vi "Main.vi"(0 "Search Bar":string, 1 "Copy":bool, 2 "Expand/Collapse All":bool, 5 "Tree":string[](tree), 7 "Top Level folder path":path, 11 "Error In":errorcluster) -> (4 "Report String":string, 15 "Error Out":errorcluster)   [LabVIEW 2019]
doc: "Implements a file explorer interface to display folders and files, displaying attributes and supporting operations like selection, copying, sorting and report generation about the folders."
uses:
  Controls/Queue Operation.ctl
  Controls/Queue Element.ctl
  Controls/File explorer Data.ctl
  Controls/Item.ctl
  <vilib>/Utility/miscctls.llb/LVPoint32TypeDef.ctl
panel:
  # "Instructions:\n1. Run the VI.\n2. Specify the top-level folder path and view the folder structure along with its attributes in the tree control.\n3. Tree headers acts as sorting triggers.\n4. Click the checkbox next to folder to select or deselect it. View the generated report for the checked folders in the report string.\n5. Press the Expand/Collapse button to expand/collapse all the items in the tree.\n6. Enter the folder name in the search bar to expand all the nodes that match the searched keyword.\n7. Select the files and click on the copy to copy the files in the new folder of the desired destination.\n8. Click Panel Close to stop the VI."
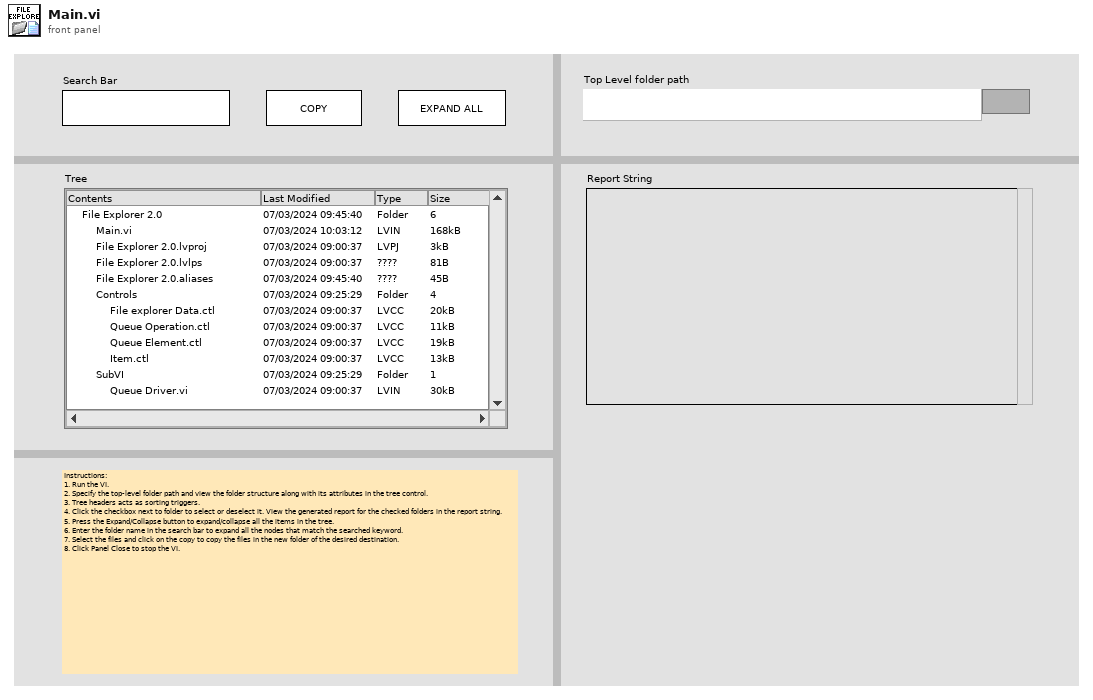
[diagram p1: front panel]
types:
  T1 = typedef "Queue Element.ctl" = cluster{"State":string, "Data":variant}
  T2 = typedef "File explorer Data.ctl" = cluster{"Path In":path, "Indent":i32, "All Folders":path[], "All Files":path[], "Folder Items":cluster{"Left Cell String":string, "Child Text":string[], "Child Tag":string, "Item Indent":i32, "Child Only?":bool, "Glyph Index":i32}[], "File Items":T3[], "Selected tags":string[], "Report String":string, "Search String":string, "Search Results":string[], "Checked Folders":string[], "Files Selected":string[], "Stop Event":refnum<user-event>, "Sort Header":i32, "Time Flag":i16, "Type Flag":i16, "Size Flag":i16, "Reverse?":bool, "New Folder Path":path, "Expand?":bool, "Open? State":bool[], "Nodes":path[]}
  T3 = typedef "Item.ctl" = cluster{"Left Cell String":string, "Child Text":string[], "Child Tag":string, "Child Only?":bool, "Parent Tag":string, "Item Indent":i32}
  T4 = typedef "Queue Operation.ctl" = enum16{"Create", "Enqueue", "Enqueue N", "Dequeue", "Enstack N", "Flush", "Release"}
  T5 = cluster{"Left Cell String":string, "Child Text":string[], "Child Tag":string, "Item Indent":i32, "Child Only?":bool, "Glyph Index":i32}
  T6 = typedef "LVPoint32TypeDef.ctl" = cluster{"Horizontal":i32, "Vertical":i32}
  T7 = cluster{"Left Cell String":string, "Child Text":string[], "Child Tag":string, "Item Indent":i32, "Child Only?":bool, "Glyph Index":i32}[]
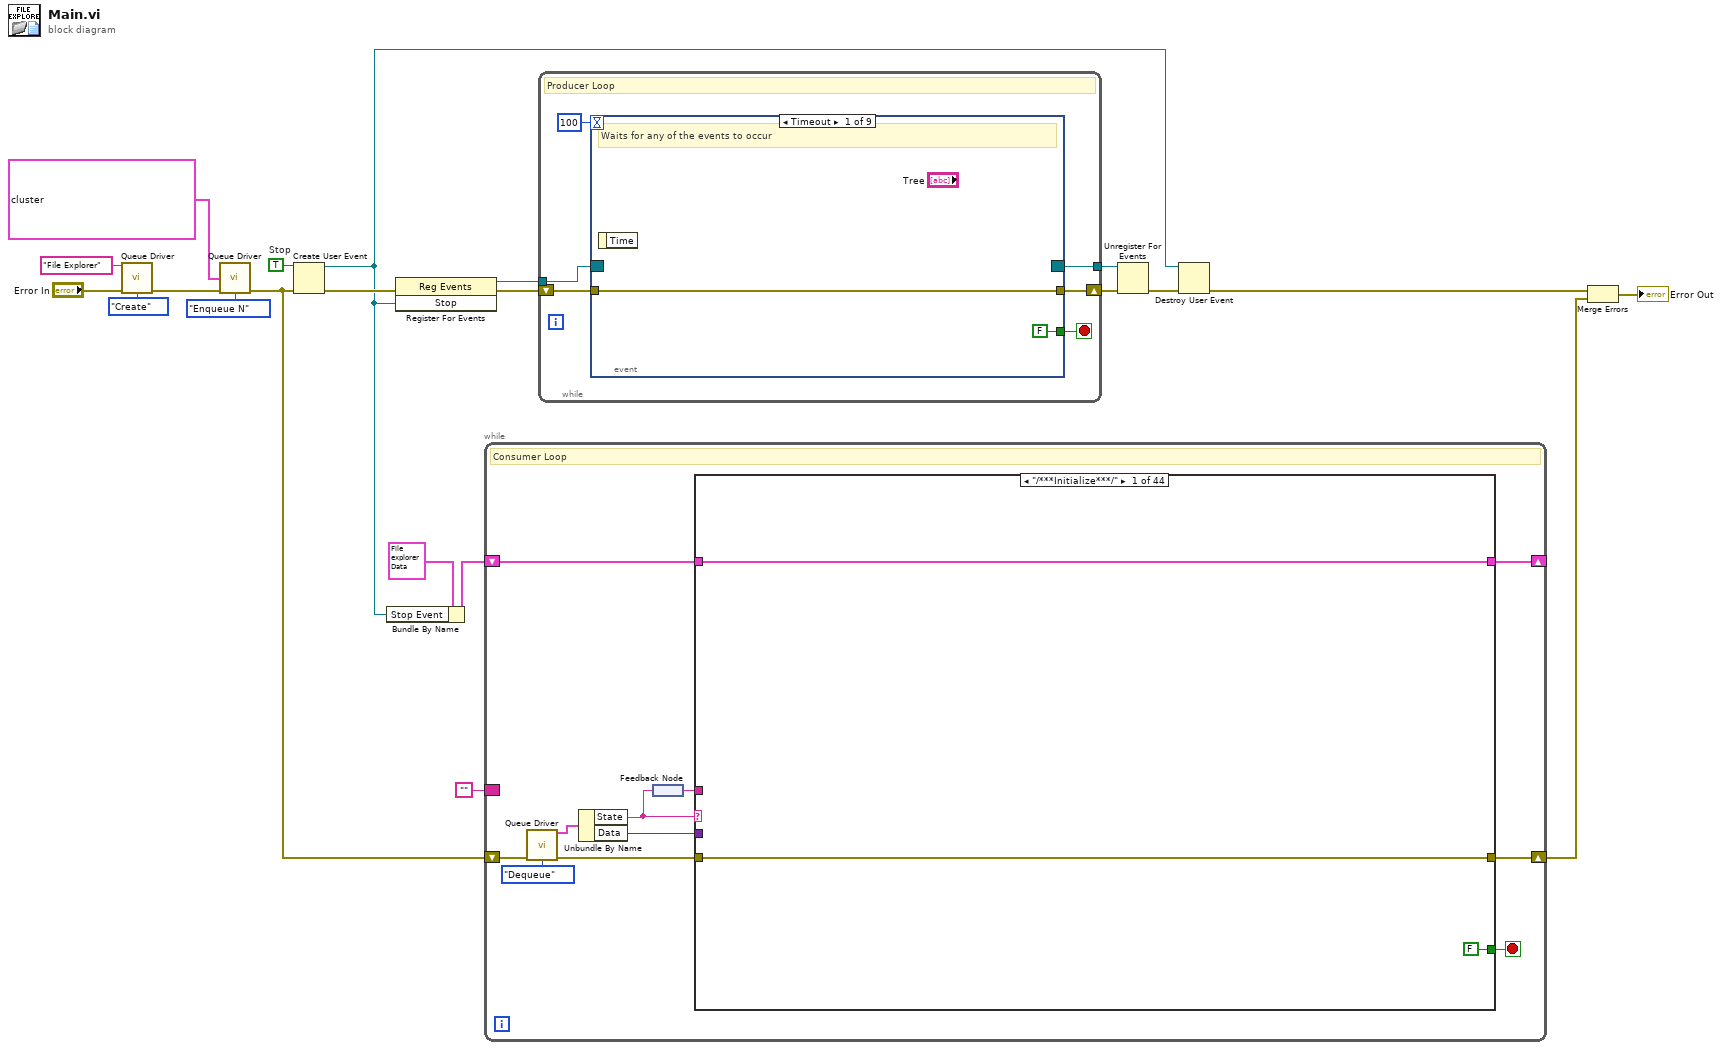
[diagram p0: block diagram]
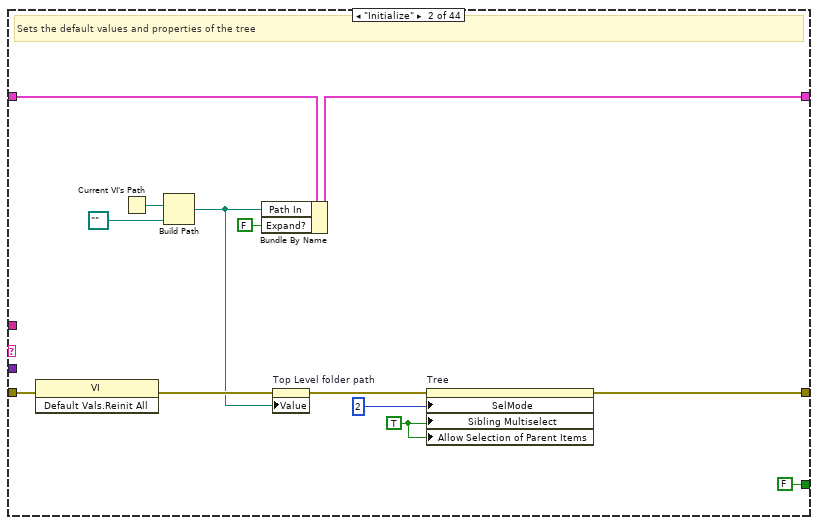
[diagram p2: hidden frame]
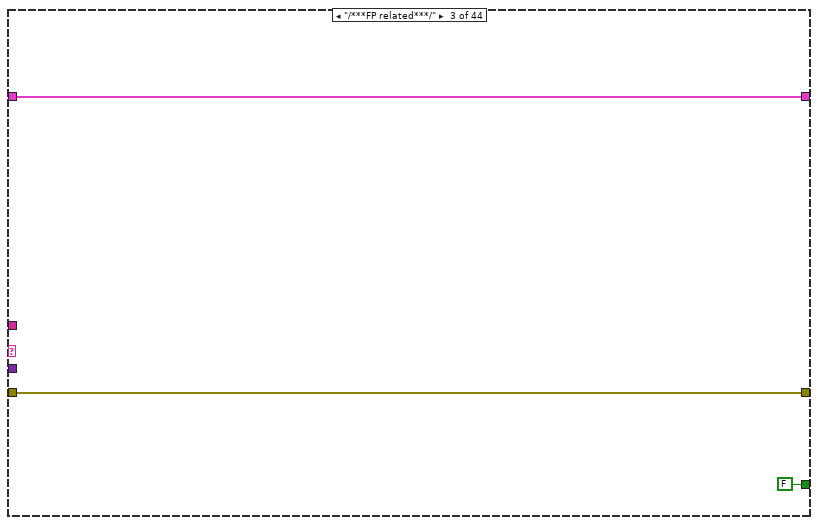
[diagram p3: hidden frame]
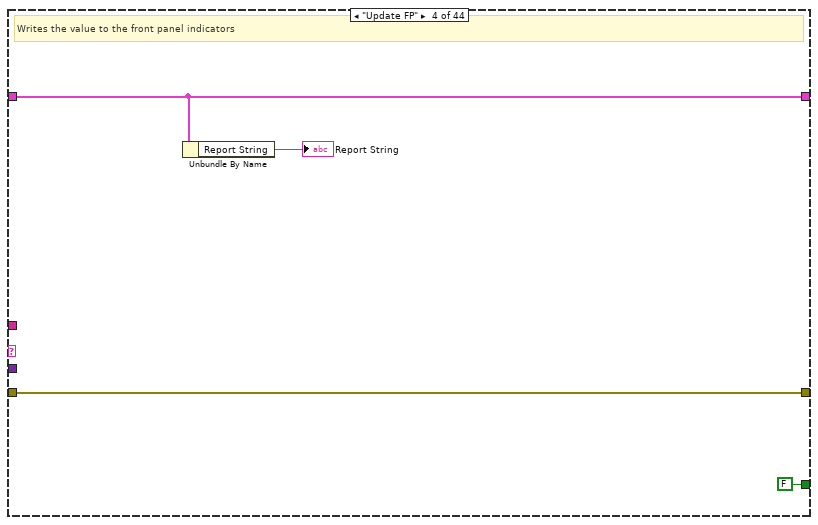
[diagram p4: hidden frame]
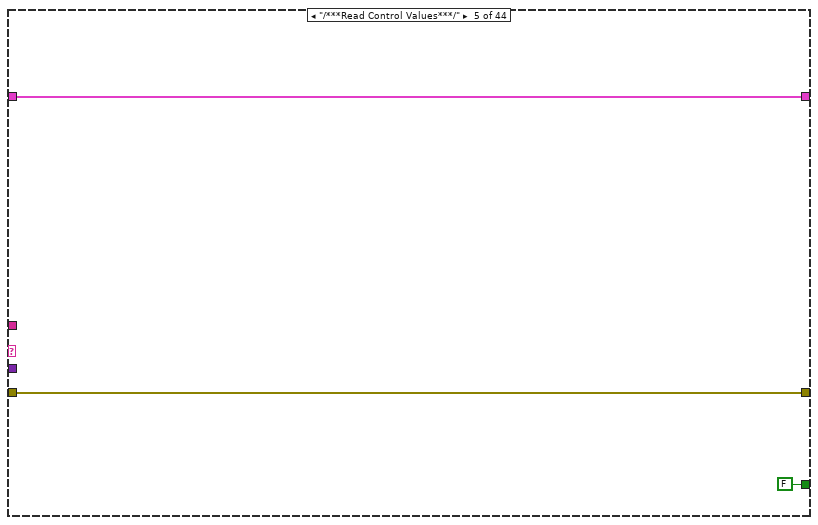
[diagram p5: hidden frame]
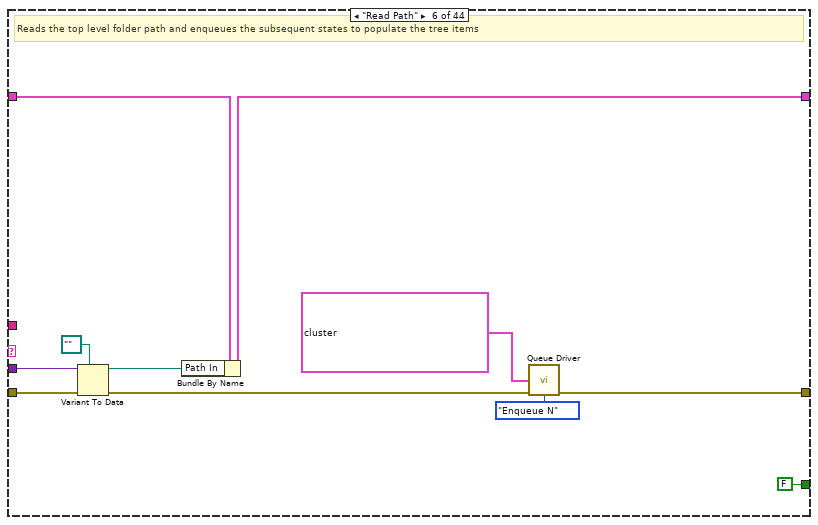
[diagram p6: hidden frame]
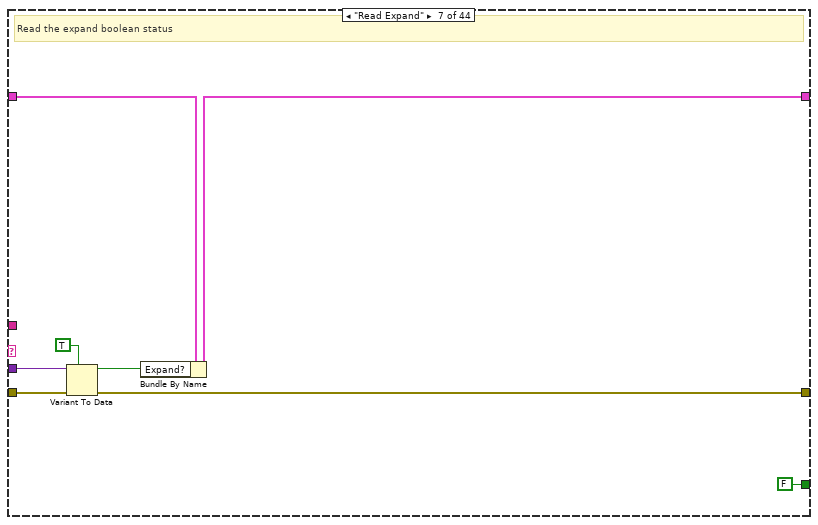
[diagram p7: hidden frame]
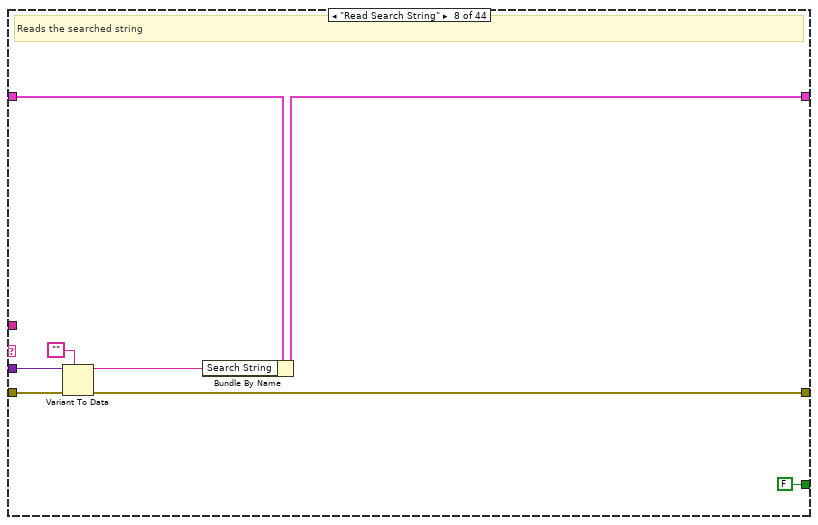
[diagram p8: hidden frame]
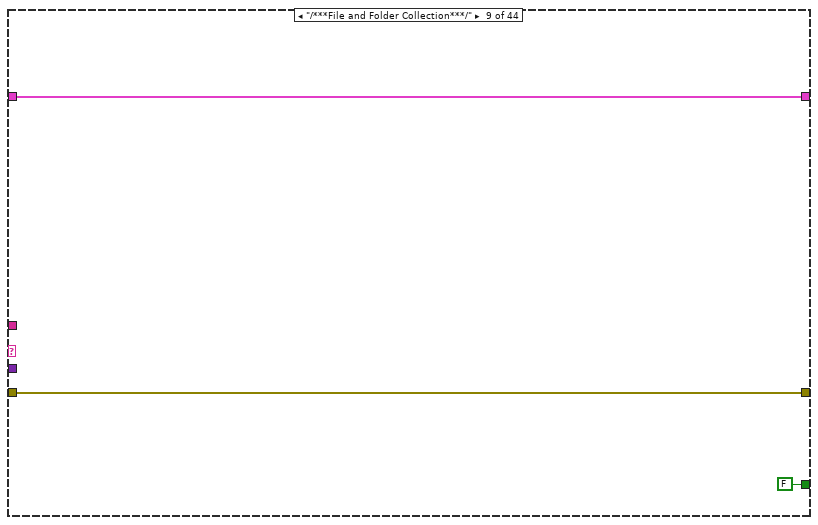
[diagram p9: hidden frame]
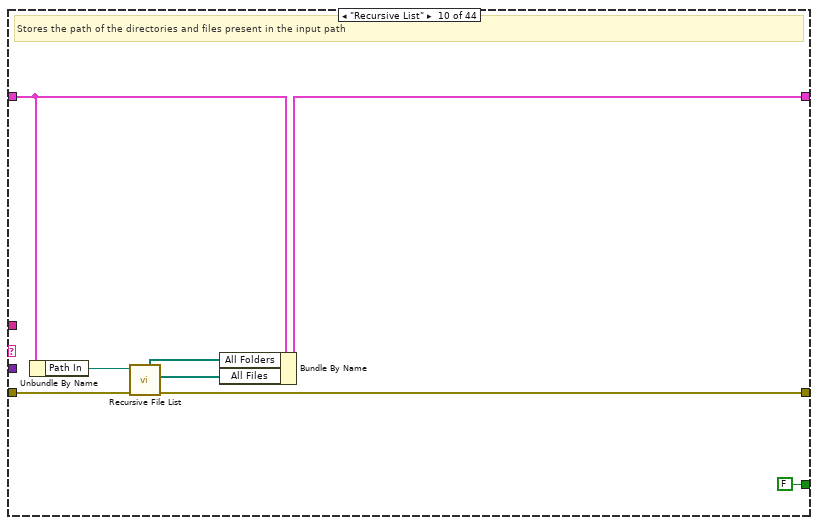
[diagram p10: hidden frame]
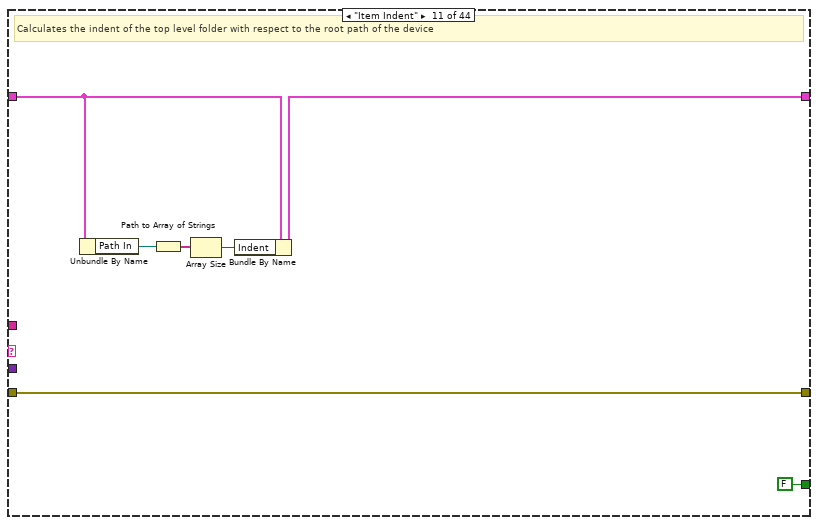
[diagram p11: hidden frame]
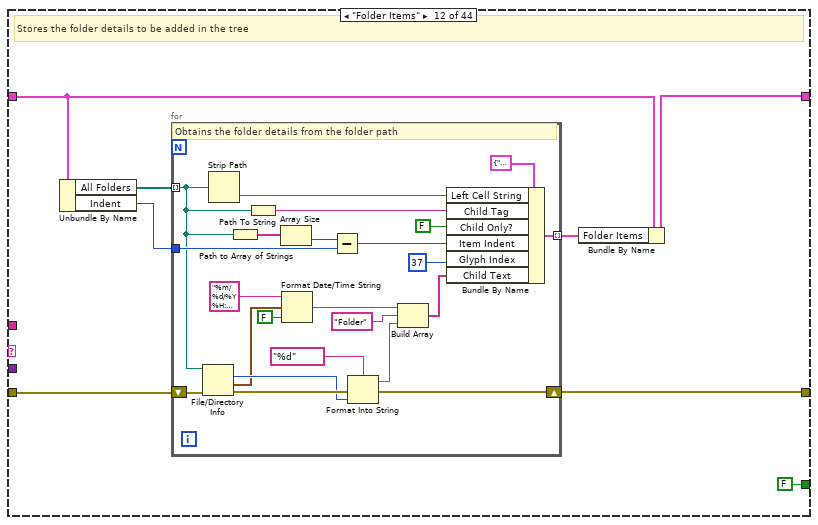
[diagram p12: hidden frame]
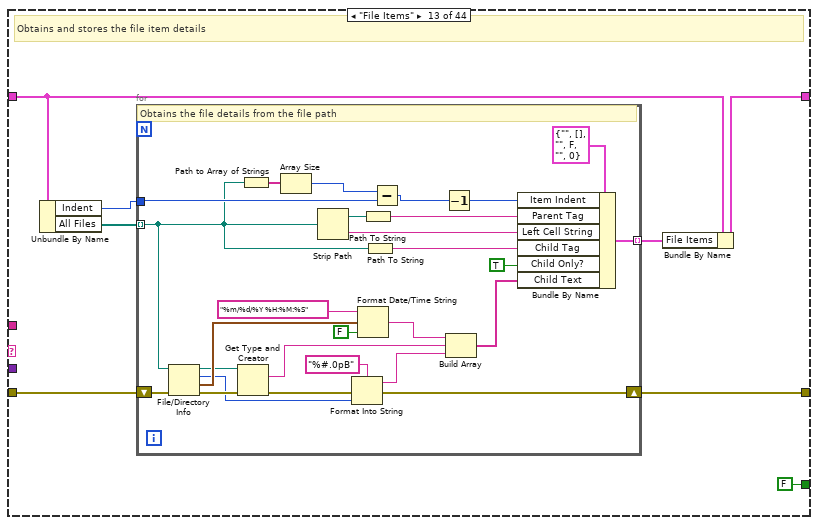
[diagram p13: hidden frame]
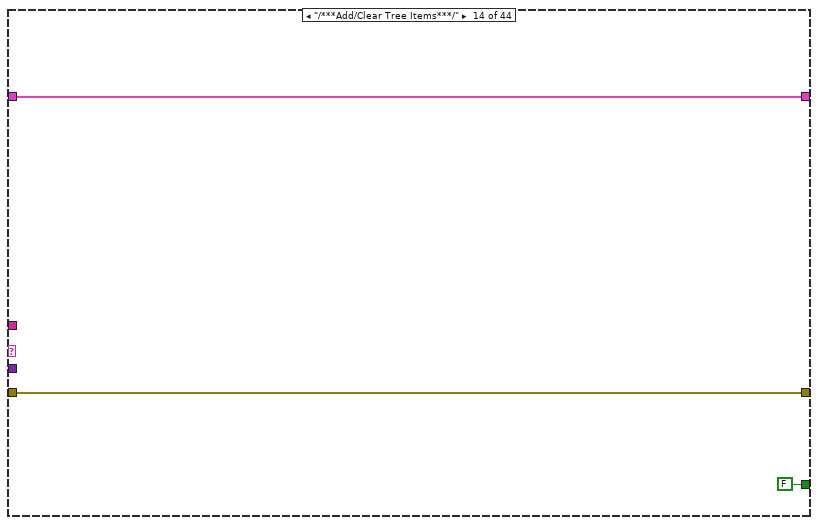
[diagram p14: hidden frame]
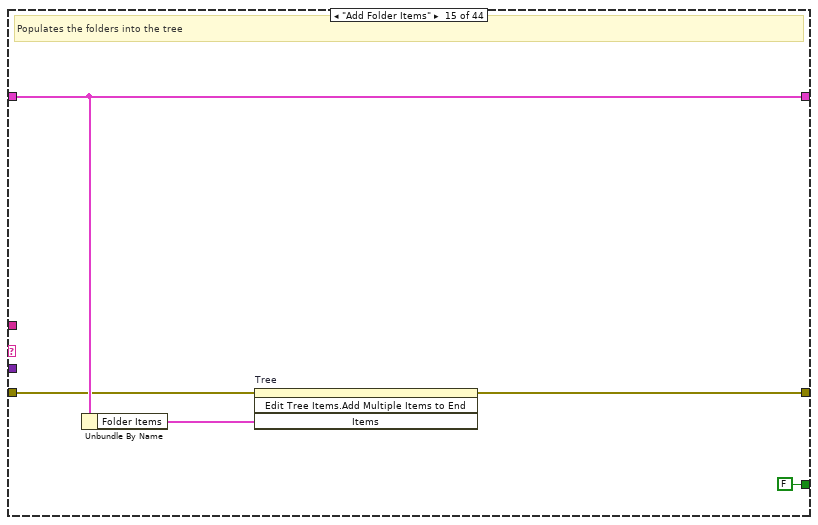
[diagram p15: hidden frame]
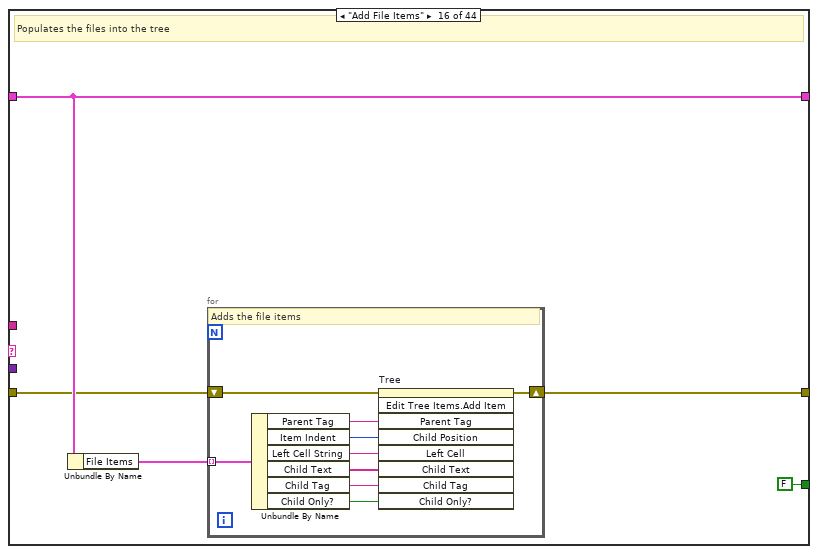
[diagram p16: hidden frame]
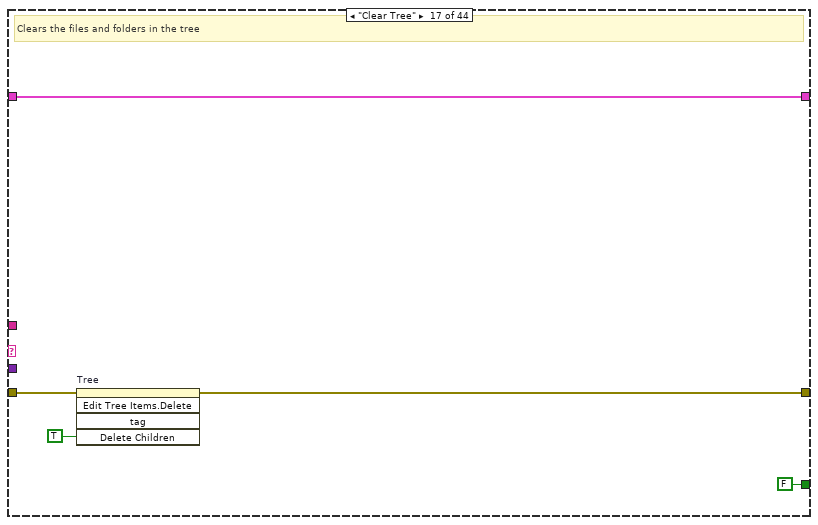
[diagram p17: hidden frame]
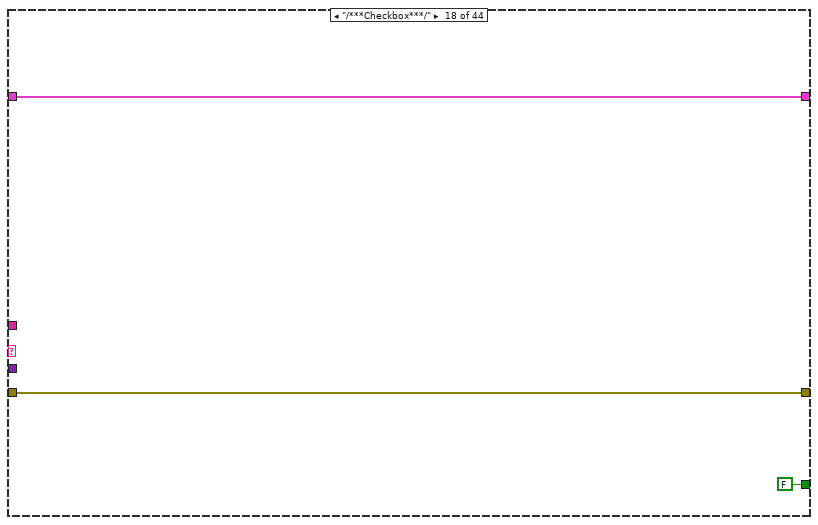
[diagram p18: hidden frame]
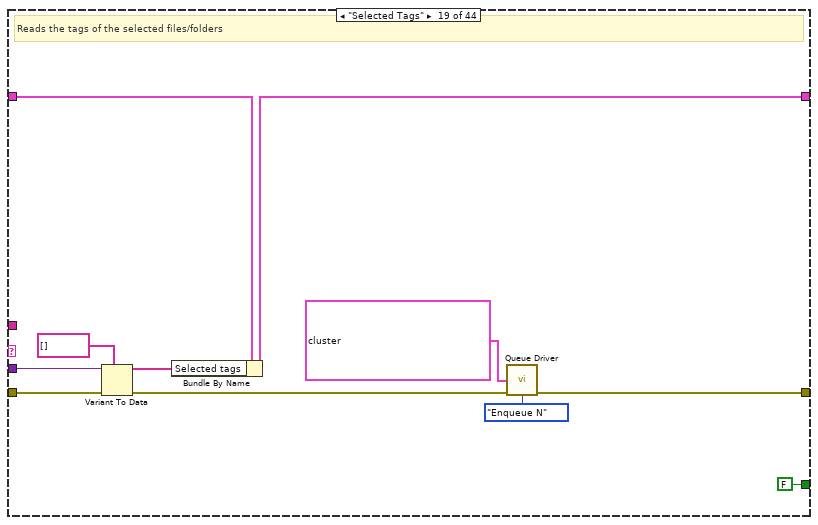
[diagram p19: hidden frame]
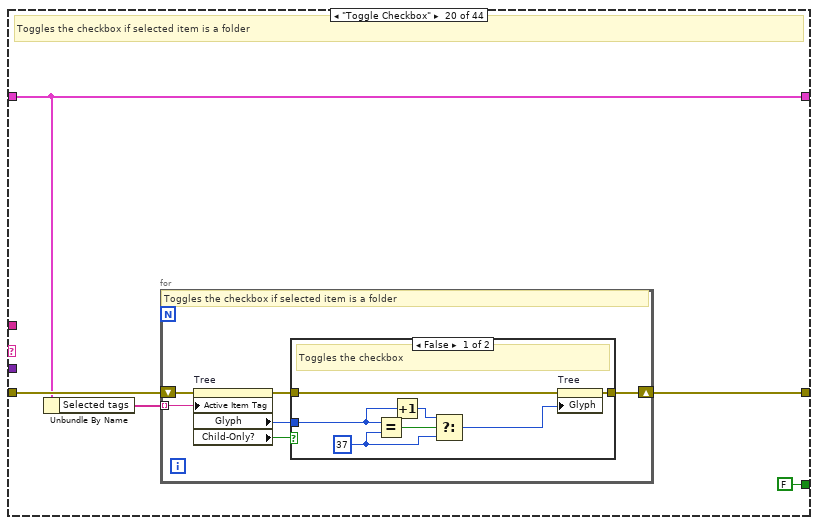
[diagram p20: hidden frame]
diagram:
  w10 = TRUE  # Stop
  n1 = call "Queue Driver.vi"("Queue Name"="File Explorer", "Error In"="Error In", "Queue Operation"=Queue_Operation."Create") -> ("Error Out"=w18:errorcluster)  [unwired: 11 in, 1 out]
  n2 = call "Queue Driver.vi"("Array of Elements"=T1[] [{"State"="Initialize", "Data"=variant}, {"State"="Clear Tree", "Data"=variant}, {"State"="Recursive List", "Data"=variant}, {"State"="Item Indent", "Data"=variant}, {"State"="Folder Items", "Data"=variant}, {"State"="File Items", "Data"=variant}, {"State"="Add Folder Items", "Data"=variant}, {"State"="Expand or Collapse", "Data"=variant}, {"State"="Add File Items", "Data"=variant}], "Error In"=w18, "Queue Operation"=Queue_Operation."Enqueue N") -> ("Error Out"=w4:errorcluster)  [unwired: 11 in, 1 out]
  n3 = Create User Event(user event datatype=w10, error in=w4) -> (user event=w2:refnum<user-event>, error out=w11:errorcluster)
  n4 = Bundle By Name(cluster=T2 {"Path In"=path "", "Indent"=0, "All Folders"=[], "All Files"=[], "Folder Items"=[], "File Items"=[], "Selected tags"=[], "Report String"="", "Search String"="", "Search Results"=[], "Checked Folders"=[], "Files Selected"=[], "Stop Event"=refnum, "Sort Header"=0, "Time Flag"=0, "Type Flag"=0, "Size Flag"=0, "Reverse?"=TRUE, "New Folder Path"=path "", "Expand?"=TRUE, "Open? State"=[], "Nodes"=[]}, "Stop Event"=w2) -> (w3:T2)
  n5 = register-events(error in=w11, w2) -> (reference out=w9:refnum<event-registration>, error out=w21:errorcluster)  [unwired: 1 in]
  n6 = while {
    border: "" ("State") -> [_]
    shift-right: [w32] -> w12
    shift-left: w4 -> [w31]
    shift-right: [w24] -> _
    shift-left: w3 -> [w25]
    stop <- w23 stop-if-true
    # "Consumer Loop"
    n7 = call "Queue Driver.vi"("Error In"=w31, "Queue Operation"=Queue_Operation."Dequeue") -> ("Dequeue Element"=w22:T1, "Error Out"=w30:errorcluster)  [unwired: 12 in]
    n8 = Unbundle By Name(w22) -> ("State"=w28:string, "Data"=w29:variant)
    n9 = feedback-in #1(w28) -> ()
    n10 = feedback #1() -> (w27:string)
    n11 = case shown="\"/***Initialize***/\"" w28 {
      tunnel: w30 -> [w35 w48 w51 w55 w58 w69 w76 w85 w88 w94 w103 w108 w141 w172 w176 w181 w196 w199 w210 w214 w232 w238 w251 w271 w275 w289 w300 w304 w319 w332 w372 w382 w397 w420 w454 w457 w465 w473 w485 w488 w496 w514 w520 w525]
      tunnel: [w35 w46 w51 w55 w58 w60 w75 w83 w88 w91 w103 w107 w140 w172 w175 w180 w194 w199 w202 w215 w232 w239 w250 w271 w274 w292 w300 w303 w317 w331 w366 w382 w386 w410 w453 w457 w464 w476 w484 w488 w492 w514 w518 w525] -> w32
      tunnel: w29 -> [_ _ _ _ _ w67 w74 w82 _ _ _ _ _ _ _ _ _ _ w209 _ _ _ _ _ _ _ _ _ _ _ _ _ w396 w418 _ _ _ _ _ _ _ _ _ _]
      tunnel: w27 -> [_ _ _ _ _ _ _ _ _ _ _ _ _ _ _ _ _ _ _ _ _ _ _ _ _ _ _ _ _ _ _ _ _ _ _ _ _ _ _ _ w495 _ _ _]
      tunnel: w25 -> [w34 w47 w50 w54 w57 w68 w77 w84 w87 w96 w102 w105 w142 w171 w177 w182 w195 w198 w206 w213 w231 w237 w255 w270 w279 w291 w299 w307 w318 w327 w374 w381 w392 w415 w450 w456 w463 w475 w483 w487 w491 w513 w521 w523]
      tunnel: [w34 w43 w50 w54 w57 w65 w72 w80 w87 w93 w99 w104 w139 w171 w177 w182 w195 w198 w207 w213 w231 w235 w253 w270 w277 w291 w299 w307 w315 w326 w374 w381 w392 w416 w450 w456 w461 w475 w483 w487 w491 w513 w521 w523] -> w24
      tunnel: [FALSE FALSE FALSE FALSE FALSE FALSE FALSE FALSE FALSE FALSE FALSE FALSE FALSE FALSE FALSE FALSE FALSE FALSE FALSE FALSE FALSE FALSE FALSE FALSE FALSE FALSE FALSE FALSE FALSE FALSE FALSE FALSE FALSE FALSE FALSE FALSE FALSE FALSE FALSE FALSE FALSE FALSE TRUE FALSE] -> w23
      frame "/***Initialize***/" {
      }
      frame "Initialize" {
        w44 = TRUE ("Sibling Multiselect")
        # "Sets the default values and properties of the tree"
        n12 = invoke on="Invoke Node" class="VI" method="Default Vals.Reinit All"(error in=w48) -> (error out=w40:errorcluster)  [unwired: 2 in, 2 out]
        n13 = Current VI's Path() -> (path=w42:path)
        n14 = Build Path(base path=w42, name or relative path=path "..") -> (appended path=w38:path)
        n15 = Bundle By Name(cluster=w47, "Path In"=w38, "Expand?"=FALSE) -> (w43:T2)
        n16 = property on="Top Level folder path" class="Path"(error in=w40, "Value"=w38) -> (error out=w39:errorcluster)  [unwired: 1 in, 1 out]
        n17 = property on="Tree" class="Tree (strict)"(error in=w39, "SelMode"=2 ("Selection Mode"), "Sibling Multiselect"=w44, "Allow Selection of Parent Items"=w44) -> (error out=w46:errorcluster)  [unwired: 1 in, 1 out]
      }
      frame "/***FP related***/" {
      }
      frame "Update FP" {
        # "Writes the value to the front panel indicators"
        n18 = Unbundle By Name(w54) -> ("Report String"=→"Report String":string)
      }
      frame "/***Read Control Values***/" {
      }
      frame "Read Path" {
        # "Reads the top level folder path and enqueues the subsequent states to populate the tree items"
        n19 = Variant To Data(error in=w69, type=path "", Variant=w67) -> (data=w64:path, error out=w61:errorcluster)
        n20 = Bundle By Name(cluster=w68, "Path In"=w64) -> (w65:T2)
        n21 = call "Queue Driver.vi"("Array of Elements"=T1[] [{"State"="Clear Tree", "Data"=variant}, {"State"="Recursive List", "Data"=variant}, {"State"="Item Indent", "Data"=variant}, {"State"="Folder Items", "Data"=variant}, {"State"="File Items", "Data"=variant}, {"State"="Add Folder Items", "Data"=variant}, {"State"="Expand or Collapse", "Data"=variant}, {"State"="Add File Items", "Data"=variant}], "Error In"=w61, "Queue Operation"=Queue_Operation."Enqueue N") -> ("Error Out"=w60:errorcluster)  [unwired: 11 in, 1 out]
      }
      frame "Read Expand" {
        # "Read the expand boolean status"
        n22 = Variant To Data(error in=w76, type=TRUE, Variant=w74) -> (data=w71:bool, error out=w75:errorcluster)
        n23 = Bundle By Name(cluster=w77, "Expand?"=w71) -> (w72:T2)
      }
      frame "Read Search String" {
        # "Reads the searched string"
        n24 = Variant To Data(error in=w85, type="" ("Search Bar"), Variant=w82) -> (data=w79:string, error out=w83:errorcluster)
        n25 = Bundle By Name(cluster=w84, "Search String"=w79) -> (w80:T2)
      }
      frame "/***File and Folder Collection***/" {
      }
      frame "Recursive List" {
        # "Stores the path of the directories and files present in the input path"
        n26 = Unbundle By Name(w96) -> ("Path In"=w95:path)
        n27 = call <vilib>:"Recursive File List.vi"("error in (no error)"=w94, "Folder Path"=w95) -> ("error out"=w91:errorcluster, "All Files in Dir"=w92:path[], "All Folders"=w89:path[])  [unwired: 5 in, 2 out]
        n28 = Bundle By Name(cluster=w96, "All Folders"=w89, "All Files"=w92) -> (w93:T2)
      }
      frame "Item Indent" {
        # "Calculates the indent of the top level folder with respect to the root path of the device"
        n29 = Unbundle By Name(w102) -> ("Path In"=w101:path)
        n30 = Path to Array of Strings(0:w101) -> (2:w100:string[])  [unwired: 1 out]
        n31 = Array Size(array=w100) -> (size(s)=w98:i32)
        n32 = Bundle By Name(cluster=w102, "Indent"=w98) -> (w99:T2)
      }
      frame "Folder Items" {
        # "Stores the folder details to be added in the tree"
        n33 = Unbundle By Name(w105) -> ("All Folders"=w111:path[], "Indent"=w110:i32)
        n34 = for {
          tunnel: [w132] -> w109 mode=indexing
          tunnel: w111 -> [w112] mode=indexing
          tunnel: w110 -> [w128]
          shift-right: [w119] -> w107
          shift-left: w108 -> [w120]
          # "Obtains the folder details from the folder path"
          n35 = File/Directory Info(path=w112, error in=w120) -> (size=w126:i64, last mod=w123:timestamp, error out=w127:errorcluster)  [unwired: 4 out]
          n36 = Strip Path(path=w112) -> (name=w129:string)  [unwired: 1 out]
          n37 = Path to Array of Strings(0:w112) -> (2:w131:string[])  [unwired: 1 out]
          n38 = Path To String(path=w112) -> (string=w116:string)
          n39 = Array Size(array=w131) -> (size(s)=w130:i32)
          n40 = Format Date/Time String(time format string (%c)="%m/%d/%Y %H:%M:%S", seconds (now)=w123, UTC format=FALSE) -> (date/time string=w121:string)
          n41 = Subtract(x=w130, y=w128) -> (x-y=w115:i32)
          n42 = Format Into String(format string="%d", error in=w127, w126) -> (resulting string=w117:string, error out=w119:errorcluster)  [unwired: 1 in]
          n43 = Build Array(w121, "Folder" ("element"), w117) -> (w118:string[])
          n44 = Bundle By Name(cluster=T5 {"Left Cell String"="", "Child Text"=[], "Child Tag"="", "Item Indent"=0, "Child Only?"=FALSE, "Glyph Index"=0} ("Item"), "Left Cell String"=w129, "Child Tag"=w116, "Child Only?"=FALSE, "Item Indent"=w115, "Glyph Index"=37, "Child Text"=w118) -> (w132:T5)
        }
        n45 = Bundle By Name(cluster=w105, "Folder Items"=w109) -> (w104:T2)
      }
      frame "File Items" {
        # "Obtains and stores the file item details"
        n46 = Unbundle By Name(w142) -> ("Indent"=w136:i32, "All Files"=w138:path[])
        n47 = for {
          tunnel: [w160] -> w137 mode=indexing
          shift-right: [w154] -> w140
          shift-left: w141 -> [w169]
          tunnel: w138 -> [w145] mode=indexing
          tunnel: w136 -> [w150]
          # "Obtains the file details from the file path"
          n48 = File/Directory Info(path=w145, error in=w169) -> (path out=w146:path, size=w149:i64, last mod=w165:timestamp, error out=w168:errorcluster)  [unwired: 3 out]
          n49 = Get Type and Creator(4:w168, 7:w146) -> (0:w153:errorcluster, 2:w152:string)  [unwired: 2 out]
          n50 = Path to Array of Strings(0:w145) -> (2:w159:string[])  [unwired: 1 out]
          n51 = Array Size(array=w159) -> (size(s)=w151:i32)
          n52 = Strip Path(path=w145) -> (stripped path=w158:path, name=w161:string)
          n53 = Format Into String(format string="%#.0pB", error in=w153, w149) -> (resulting string=w148:string, error out=w154:errorcluster)  [unwired: 1 in]
          n54 = Format Date/Time String(time format string (%c)="%m/%d/%Y %H:%M:%S", seconds (now)=w165, UTC format=FALSE) -> (date/time string=w157:string)
          n55 = Path To String(path=w158) -> (string=w156:string)
          n56 = Path To String(path=w145) -> (string=w155:string)
          n57 = Subtract(x=w151, y=w150) -> (x-y=w143:i32)
          n58 = Decrement(x=w143) -> (x-1=w144:i32)
          n59 = Build Array(w157, w152, w148) -> (w147:string[])
          n60 = Bundle By Name(cluster=T3 {"Left Cell String"="", "Child Text"=[], "Child Tag"="", "Child Only?"=FALSE, "Parent Tag"="", "Item Indent"=0} ("Item"), "Item Indent"=w144, "Parent Tag"=w156, "Left Cell String"=w161, "Child Tag"=w155, "Child Only?"=TRUE, "Child Text"=w147) -> (w160:T3)
        }
        n61 = Bundle By Name(cluster=w142, "File Items"=w137) -> (w139:T2)
      }
      frame "/***Add/Clear Tree Items***/" {
      }
      frame "Add Folder Items" {
        # "Populates the folders into the tree"
        n62 = Unbundle By Name(w177) -> ("Folder Items"=w174:T7)
        n63 = invoke on="Tree" class="Tree (strict)" method="Edit Tree Items.Add Multiple Items to End"(error in=w176, "Items"=w174) -> (error out=w175:errorcluster)  [unwired: 2 in, 3 out]
      }
      frame "Add File Items" {
        # "Populates the files into the tree"
        n64 = Unbundle By Name(w182) -> ("File Items"=w179:T3[])
        n65 = for {
          shift-right: [w190] -> w180
          shift-left: w181 -> [w191]
          tunnel: w179 -> [w189] mode=indexing
          # "Adds the file items"
          n66 = Unbundle By Name(w189) -> ("Parent Tag"=w184:string, "Item Indent"=w183:i32, "Left Cell String"=w187:string, "Child Text"=w186:string[], "Child Tag"=w185:string, "Child Only?"=w188:bool)
          n67 = invoke on="Tree" class="Tree (strict)" method="Edit Tree Items.Add Item"(error in=w191, "Parent Tag"=w184, "Child Position"=w183, "Left Cell"=w187, "Child Text"=w186, "Child Tag"=w185, "Child Only?"=w188) -> (error out=w190:errorcluster)  [unwired: 2 in, 8 out]
        }
      }
      frame "Clear Tree" {
        # "Clears the files and folders in the tree"
        n68 = invoke on="Tree" class="Tree (strict)" method="Edit Tree Items.Delete"(error in=w196, "Delete Children"=TRUE ("Sibling Multiselect")) -> (error out=w194:errorcluster)  [unwired: 3 in, 4 out]
      }
      frame "/***Checkbox***/" {
      }
      frame "Selected Tags" {
        # "Reads the tags of the selected files/folders"
        n69 = Variant To Data(error in=w210, type=string[] [] ("NewVal"), Variant=w209) -> (data=w205:string[], error out=w203:errorcluster)
        n70 = Bundle By Name(cluster=w206, "Selected tags"=w205) -> (w207:T2)
        n71 = call "Queue Driver.vi"("Array of Elements"=T1[] [{"State"="Toggle Checkbox", "Data"=variant}, {"State"="Selected Files", "Data"=variant}, {"State"="Selected Folders", "Data"=variant}, {"State"="Folder Details", "Data"=variant}, {"State"="Update FP", "Data"=variant}] ("appended array"), "Error In"=w203, "Queue Operation"=Queue_Operation."Enqueue N") -> ("Error Out"=w202:errorcluster)  [unwired: 11 in, 1 out]
      }
      frame "Toggle Checkbox" {
        # "Toggles the checkbox if selected item is a folder"
        n72 = Unbundle By Name(w213) -> ("Selected tags"=w212:string[])
        n73 = for {
          shift-right: [w221] -> w215
          shift-left: w214 -> [w220]
          tunnel: w212 -> [w217] mode=indexing
          # "Toggles the checkbox if selected item is a folder"
          n74 = property on="Tree" class="Tree (strict)"(error in=w220, "Active Item Tag"=w217) -> (error out=w219:errorcluster, "Glyph"=w218:i32, "Child-Only?"=w216:bool)  [unwired: 1 in, 1 out]
          n75 = case shown="False" w216 {
            tunnel: [w228 w229] -> w221
            tunnel: w219 -> [w227 w229]
            tunnel: w218 -> [w222 _]
            frame False {
              w224 = 37 ("x")
              # "Toggles the checkbox"
              n76 = Equal?(x=w222, y=w224) -> (x = y?=w225:bool)
              n77 = Increment(x=w222) -> (x+1=w223:i32)
              n78 = Select(t=w223, s=w225, f=w224) -> (s? t:f=w226:i32)
              n79 = property on="Tree" class="Tree (strict)"(error in=w227, "Glyph"=w226) -> (error out=w228:errorcluster)  [unwired: 1 in, 1 out]
            }
            frame True {
            }
          }
        }
      }
      frame "/***Report Generation***/" {
      }
      frame "Selected Folders" {
        # "Stores the folders in which checkbox is ticked"
        n80 = Unbundle By Name(w237) -> ("All Folders"=w236:path[])
        n81 = for {
          shift-right: [w246] -> w239
          shift-left: w238 -> [w247]
          tunnel: w236 -> [w245] mode=indexing
          tunnel: [w242] -> w233 mode=indexing if=w243
          # "separates the checked folders based on the symbol index"
          n82 = Path To String(path=w245) -> (string=w244:string)
          n83 = property on="Tree" class="Tree (strict)"(error in=w247, "Active Item Tag"=w244) -> (error out=w246:errorcluster, "Active Item Tag"=w242:string, "Glyph"=w241:i32)  [unwired: 1 in, 1 out]
          n84 = Equal?(x=w241, y=38 ("x")) -> (x = y?=w243:bool)
        }
        n85 = Bundle By Name(cluster=w237, "Checked Folders"=w233) -> (w235:T2)
      }
      frame "Folder Details" {
        # "Obtains the details of the checked folders and prepares the report string"
        n86 = Unbundle By Name(w255) -> ("Checked Folders"=w254:string[])
        n87 = for {
          tunnel: w254 -> [w262] mode=indexing
          shift-right: [w266] -> w250
          shift-left: w251 -> [w268]
          tunnel: [w260] -> w249 mode=indexing
          w258 = 1 ("Active Cell:Active Column Number")
          # "Prepares the report string for the checked folders"
          n88 = Increment(x=w258) -> (x+1=w256:i32)
          n89 = Increment(x=w256) -> (x+1=w257:i32)
          n90 = property on="Tree" class="Tree (strict)"(error in=w268, "Active Item Tag"=w262, "ActiveColNum"=w258, "ActiveColNum"=w256, "ActiveColNum"=w257) -> (error out=w267:errorcluster, "Active Item Tag"=w261:string, "Cell String"=w265:string, "Cell String"=w264:string, "Cell String"=w263:string)  [unwired: 1 in, 1 out]
          n91 = Format Into String(format string="Path: %s \nLast Modified: %s\nType: %s\nSize: %s\n<------------------------------------------------------------------------>\\n", error in=w267, w261, w265, w264, w263) -> (resulting string=w260:string, error out=w266:errorcluster)  [unwired: 1 in]
        }
        n92 = Concatenate Strings(w249) -> (w252:string)
        n93 = Bundle By Name(cluster=w255, "Report String"=w252) -> (w253:T2)
      }
      frame "/***Search Operation***/" {
      }
      frame "Search Results" {
        # "Extracts the tags of the folders who match with the search string"
        n94 = Unbundle By Name(w279) -> ("Folder Items"=w278:T7, "Search String"=w273:string)
        n95 = for {
          tunnel: w278 -> [w287] mode=indexing
          tunnel: [w285] -> w276 mode=indexing if=w286
          tunnel: w273 -> [w283]
          shift-right: [w282] -> w274
          shift-left: w275 -> [w282]
          # "Extracts the tag if folder name matches with search string"
          n96 = Unbundle By Name(w287) -> ("Child Tag"=w285:string, "Left Cell String"=w284:string)
          n97 = To Lower Case(string=w283) -> (all lower case string=w280:string)
          n98 = To Lower Case(string=w284) -> (all lower case string=w281:string)
          n99 = Equal?(x=w281, y=w280) -> (x = y?=w286:bool)
        }
        n100 = Bundle By Name(cluster=w279, "Search Results"=w276) -> (w277:T2)
      }
      frame "Expand Search" {
        # "Makes the searched folder visible and open in the tree"
        n101 = Unbundle By Name(w291) -> ("Search Results"=w290:string[])
        n102 = for {
          shift-right: [w297] -> w292
          shift-left: w289 -> [w295]
          tunnel: w290 -> [w293] mode=indexing
          # "Makes the folder visible and open"
          n103 = invoke on="Tree" class="Tree (strict)" method="Open/Close.Ensure Visible"(error in=w295, "tag"=w293) -> (error out=w294:errorcluster)  [unwired: 2 in, 3 out]
          n104 = invoke on="Tree" class="Tree (strict)" method="Open/Close.Item"(error in=w294, "tag"=w293, "Open"=TRUE ("Open?")) -> (error out=w297:errorcluster)  [unwired: 2 in, 4 out]
        }
      }
      frame "/***Copy Opearation***/" {
      }
      frame "Trigger Copy" {
        # "Triggers the copy operation if any of the files is selected"
        n105 = Unbundle By Name(w307) -> ("Files Selected"=w306:string[])
        n106 = Array Size(array=w306) -> (size(s)=w305:i32)
        n107 = Not Equal To 0?(x=w305) -> (x != 0?=w302:bool)
        n108 = case shown="True" w302 {
          tunnel: [w308 w310] -> w303
          tunnel: w304 -> [w308 w311]
          frame False {
            # "No files are selected"
          }
          frame True {
            # "Files selected"
            n109 = call "Queue Driver.vi"("Array of Elements"=T1[] [{"State"="Copy Files", "Data"=variant}, {"State"="Repopulate Tree", "Data"=variant}], "Error In"=w311, "Queue Operation"=Queue_Operation."Enqueue N") -> ("Error Out"=w310:errorcluster)  [unwired: 11 in, 1 out]
          }
        }
      }
      frame "Selected Files" {
        # "Separates the selected files"
        n110 = Unbundle By Name(w318) -> ("Selected tags"=w316:string[])
        n111 = for {
          tunnel: w316 -> [w322] mode=indexing
          shift-right: [w323] -> w317
          shift-left: w319 -> [w324]
          tunnel: [w320] -> w314 mode=indexing if=w321
          # "Checks id the selected items are files and store it"
          n112 = property on="Tree" class="Tree (strict)"(error in=w324, "Active Item Tag"=w322) -> (error out=w323:errorcluster, "Active Item Tag"=w320:string, "Child-Only?"=w321:bool)  [unwired: 1 in, 1 out]
        }
        n113 = Bundle By Name(cluster=w318, "Files Selected"=w314) -> (w315:T2)
      }
      frame "Copy Files" {
        # "Copies the files in the destination selected by the user"
        n114 = call "File Dialog"("error in"=w332) -> ("selected path"=w330:path, "exists"=w329:bool, "cancelled"=w328:bool, "error out"=w333:errorcluster)  [unwired: 11 in]
        n115 = case shown="True" w328 {
          tunnel: w333 -> [w342 w361]
          tunnel: [w339 w359] -> w331
          tunnel: w330 -> [w334 _]
          tunnel: w329 -> [w341 _]
          tunnel: [w336 w363] -> w326
          tunnel: w327 -> [w337 w363]
          frame False {
            # "Checks if the path specified by user exists and creates the folder accordingly to perform copy operation"
            n116 = case shown="True" w341 {
              tunnel: w342 -> [w351 w357]
              tunnel: [w350 w356] -> w340
              tunnel: w334 -> [w349 w353]
              tunnel: [w348 w355] -> w335
              frame False {
                # "New folder created"
                n117 = Create Folder(path (use dialog)=w349, error in=w351) -> (created path=w348:path, error out=w350:errorcluster)  [unwired: 1 in, 1 out]
              }
              frame True {
                # "Given folder name already exists"
                n118 = Strip Path(path=w353) -> (name=w352:string)  [unwired: 1 out]
                n119 = Build Path(base path=w353, name or relative path=w352) -> (appended path=w354:path)
                n120 = Create Folder(path (use dialog)=w354, error in=w357) -> (created path=w355:path, error out=w356:errorcluster)  [unwired: 1 in, 1 out]
              }
            }
            n121 = Bundle By Name(cluster=w337, "New Folder Path"=w334) -> (w336:T2)
            n122 = Unbundle By Name(w336) -> ("Files Selected"=w338:string[])
            n123 = for {
              shift-right: [w345] -> w339
              shift-left: w340 -> [w346]
              tunnel: w338 -> [w347] mode=indexing
              tunnel: w335 -> [w344]
              # "Copies the selected files"
              n124 = String To Path(string=w347) -> (path=w343:path)
              n125 = Copy(8:w346, 10:w344, 11:w343) -> (0:w345:errorcluster)  [unwired: 2 in, 2 out]
            }
          }
          frame True {
            # "User cancelled the File dialog, notifies and clear the error"
            n126 = call <vilib>:"Clear Errors.vi"("error in (no error)"=w361, "specific error code to clear (0: all)"=43) -> ("error out"=w359:errorcluster)  [unwired: 4 in, 1 out]
            n127 = One Button Dialog(message="Copy operation cancelled by user.", button name ("OK")="Ok") -> ()  [unwired: 1 out]
          }
        }
      }
      frame "Repopulate Tree" {
        # "If destination path is inside the root path the tree repopulates to display the newly added folder in the tree"
        n128 = Unbundle By Name(w374) -> ("New Folder Path"=w365:path, "Path In"=w373:path)
        n129 = Path To String(path=w365) -> (string=w367:string)
        n130 = Path To String(path=w373) -> (string=w371:string)
        n131 = Search and Replace String(input string=w367, search string=w371, error in=w372) -> (number of replacements=w368:i32, error out=w369:errorcluster)  [unwired: 5 in, 2 out]
        n132 = Greater Than 0?(x=w368) -> (x > 0?=w370:bool)
        n133 = case shown="True" w370 {
          tunnel: w369 -> [w375 w378]
          tunnel: [w375 w377] -> w366
          frame False {
          }
          frame True {
            # "Repopulates the tree"
            n134 = call "Queue Driver.vi"("Array of Elements"=T1[] [{"State"="Save Node Status", "Data"=variant}, {"State"="Clear Tree", "Data"=variant}, {"State"="Recursive List", "Data"=variant}, {"State"="Folder Items", "Data"=variant}, {"State"="File Items", "Data"=variant}, {"State"="Add Folder Items", "Data"=variant}, {"State"="Open Nodes", "Data"=variant}, {"State"="Add File Items", "Data"=variant}], "Error In"=w378, "Queue Operation"=Queue_Operation."Enqueue N") -> ("Error Out"=w377:errorcluster)  [unwired: 11 in, 1 out]
          }
        }
      }
      frame "/***Sort Operation***/" {
      }
      frame "Trigger Sort" {
        # "Checks if the mouse down is to trigger sort"
        n135 = Variant To Data(error in=w397, type=T6 {"Horizontal"=0, "Vertical"=0} ("Coords"), Variant=w396) -> (data=w393:T6, error out=w394:errorcluster)
        n136 = invoke on="Tree" class="Tree (strict)" method="Point To Row Column"(error in=w394, "Point"=w393) -> (error out=w387:errorcluster, "Tag"=w391:string, "Col"=w384:i32)  [unwired: 6 in, 5 out]
        n137 = Not Equal To 0?(x=w384) -> (x != 0?=w388:bool)
        n138 = Equal?(x="TREE_COLUMN_HEADERS", y=w391) -> (x = y?=w389:bool)
        n139 = And(x=w389, y=w388) -> (x .and. y?=w385:bool)
        n140 = case shown="True" w385 {
          tunnel: w387 -> [w398 w407]
          tunnel: [w398 w406] -> w386
          tunnel: w384 -> [_ w400]
          frame False {
            # "Header to trigger sort is not clicked"
          }
          frame True {
            # "Triggers the Sort"
            n141 = To Variant(anything=w400) -> (Variant=w404:variant)
            n142 = Bundle By Name(cluster=T1 {"State"="", "Data"=variant} ("Enqueue Element"), "Data"=w404, "State"="Sort Type") -> (w405:T1)
            n143 = Build Array(w405, T1 {"State"="Sort", "Data"=variant} ("element")) -> (w401:T1[])
            n144 = call "Queue Driver.vi"("Array of Elements"=w401, "Error In"=w407, "Queue Operation"=Queue_Operation."Enqueue N") -> ("Error Out"=w406:errorcluster)  [unwired: 11 in, 1 out]
          }
        }
      }
      frame "Sort Type" {
        # "Decides the type of sort to be performed"
        n145 = Variant To Data(error in=w420, type=0 ("Case Sensitivity"), Variant=w418) -> (data=w417:i32, error out=w411:errorcluster)
        n146 = Unbundle By Name(w415) -> ("Time Flag"=w414:i16, "Type Flag"=w413:i16, "Size Flag"=w412:i16)
        n147 = case shown="2" w417 {
          selector: w417 -> [_ w426 w435 w443]
          tunnel: [w422 w429 w437 w445] -> w416
          tunnel: w415 -> [w422 w430 w438 w446]
          tunnel: w414 -> [_ _ w431 _]
          tunnel: w413 -> [_ _ _ w439]
          tunnel: w412 -> [_ w427 _ _]
          tunnel: w411 -> [w421 w428 w436 w444]
          tunnel: [w421 w428 w436 w444] -> w410
          frame Default {
          }
          frame 3 {
            # "Size sort"
            n148 = Not Equal To 0?(x=w427) -> (x != 0?=w423:bool)
            n149 = Not(x=w423) -> (.not. x?=w424:bool)
            n150 = Boolean To (0,1)(Boolean=w424) -> (0, 1=w425:i16)
            n151 = Bundle By Name(cluster=w430, "Reverse?"=w423, "Size Flag"=w425, "Sort Header"=w426) -> (w429:T2)
          }
          frame 1 {
            # "Last modified Sort"
            n152 = Not Equal To 0?(x=w431) -> (x != 0?=w434:bool)
            n153 = Not(x=w434) -> (.not. x?=w432:bool)
            n154 = Boolean To (0,1)(Boolean=w432) -> (0, 1=w433:i16)
            n155 = Bundle By Name(cluster=w438, "Reverse?"=w434, "Time Flag"=w433, "Sort Header"=w435) -> (w437:T2)
          }
          frame 2 {
            # "File type sort"
            n156 = Not Equal To 0?(x=w439) -> (x != 0?=w442:bool)
            n157 = Not(x=w442) -> (.not. x?=w440:bool)
            n158 = Boolean To (0,1)(Boolean=w440) -> (0, 1=w441:i16)
            n159 = Bundle By Name(cluster=w446, "Reverse?"=w442, "Type Flag"=w441, "Sort Header"=w443) -> (w445:T2)
          }
        }
      }
      frame "Sort" {
        # "Sort the contents of the tree"
        n160 = Unbundle By Name(w450) -> ("Sort Header"=w449:i32, "Reverse?"=w448:bool)
        n161 = invoke on="Tree" class="Tree (strict)" method="Edit Tree Items.Sort Children"(error in=w454, "tag"="" ("Tag"), "Sort Column"=w449, "Sort Recursively"=TRUE ("Sort Recursively?"), "Reverse Order"=w448) -> (error out=w453:errorcluster)  [unwired: 3 in, 7 out]
      }
      frame "/***Open/Close Nodes***/" {
      }
      frame "Save Node Status" {
        # "Saves the node status which will be used to repopulate the tree"
        n162 = Unbundle By Name(w463) -> ("All Folders"=w458:path[])
        n163 = Path To String(path=w458) -> (string=w462:string[])
        n164 = for {
          shift-right: [w468] -> w464
          shift-left: w465 -> [w469]
          tunnel: w462 -> [w467] mode=indexing
          tunnel: [w466] -> w460 mode=indexing
          n165 = property on="Tree" class="Tree (strict)"(error in=w469, "Active Item Tag"=w467) -> (error out=w468:errorcluster, "Open?"=w466:bool)  [unwired: 1 in, 1 out]
        }
        n166 = Bundle By Name(cluster=w463, "Nodes"=w458, "Open? State"=w460) -> (w461:T2)
      }
      frame "Open Nodes" {
        # "Open or close the node based on the saved status"
        n167 = Unbundle By Name(w475) -> ("Nodes"=w474:path[], "Open? State"=w472:bool[])
        n168 = Path To String(path=w474) -> (string=w470:string[])
        n169 = for {
          shift-right: [w480] -> w476
          shift-left: w473 -> [w479]
          tunnel: w470 -> [w478] mode=indexing
          tunnel: w472 -> [w477] mode=indexing
          # "Opens/ Closes the nodes"
          n170 = invoke on="Tree" class="Tree (strict)" method="Open/Close.Item"(error in=w479, "tag"=w478, "Open"=w477) -> (error out=w480:errorcluster)  [unwired: 2 in, 4 out]
        }
      }
      frame "Expand or Collapse" {
        # "Opens or closes all the folder"
        n171 = Unbundle By Name(w483) -> ("Expand?"=w482:bool)
        n172 = invoke on="Tree" class="Tree (strict)" method="Open/Close.Open/Close All"(error in=w485, "Open"=w482) -> (error out=w484:errorcluster)  [unwired: 2 in, 3 out]
      }
      frame "/***Error***/" {
      }
      frame "Error" {
        # "Handles the error based on user response"
        n173 = Unbundle By Name(w496) -> ("code"=w498:i32, "source"=w497:string)
        n174 = call <vilib>:"Clear Errors.vi"("error in (no error)"=w496) -> ("error out"=w503:errorcluster)  [unwired: 5 in, 1 out]
        n175 = Format Into String(format string="Error occurred in state \"%s\"!!\nError Code: %d\nError Source: %s\n\nDo you wish to continue?", error in=w503, w495, w498, w497) -> (resulting string=w501:string, error out=w493:errorcluster)  [unwired: 1 in]
        n176 = Unbundle By Name(w491) -> ("Stop Event"=w490:refnum<user-event>)
        n177 = Two Button Dialog(message=w501, 1:"Exit" ("F button name (\"Cancel\")"), 2:"Continue" ("T button name (\"OK\")")) -> (T button?=w494:bool)
        n178 = case shown="False" w494 {
          tunnel: w493 -> [w509 w511]
          tunnel: [w507 w511] -> w492
          tunnel: w490 -> [w506 _]
          frame False {
            # "Triggers to stop the VI"
            n179 = call "Queue Driver.vi"("Array of Elements"=T1[] [{"State"="Exit", "Data"=variant}], "Error In"=w509, "Queue Operation"=Queue_Operation."Enstack N") -> ("Error Out"=w510:errorcluster)  [unwired: 11 in, 1 out]
            n180 = Generate User Event(user event=w506, event data cluster=TRUE ("event data"), error in=w510) -> (error out=w507:errorcluster)  [unwired: 1 in, 1 out]
          }
          frame True {
          }
        }
      }
      frame "/***Exit***/" {
      }
      frame "Exit" {
        # "Releases the queue and stops the consumer loop"
        n181 = call "Queue Driver.vi"("Error In"=w520, "Queue Operation"=Queue_Operation."Flush") -> ("Error Out"=w519:errorcluster)  [unwired: 12 in, 1 out]
        n182 = call "Queue Driver.vi"("Error In"=w519, "Queue Operation"=Queue_Operation."Release") -> ("Error Out"=w518:errorcluster)  [unwired: 12 in, 1 out]
      }
      frame Default {
        n183 = Wait (ms)(milliseconds to wait=u32 100) -> ()  [unwired: 1 out]
      }
    }
  }
  n184 = while {
    shift-right: [w530] -> w20
    shift-left: w21 -> [w531]
    tunnel: w9 -> [w527]
    tunnel: [w526] -> w6
    stop <- w528 stop-if-true
    # "Producer Loop"
    n185 = event shown="[0] Timeout" {
      selector: w527 -> [_ _ _ _ _ _ _ _ _]
      dyn-events: [_ _ _ _ _ _ _ _ _] -> w526
      timeout: 100 -> [_ _ _ _ _ _ _ _ _]
      tunnel: w531 -> [w533 w542 w551 w555 w568 w576 w584 w592 w597]
      tunnel: [w533 w541 w550 w554 w567 w575 w583 w591 w597] -> w530
      tunnel: [FALSE ("Stop") FALSE ("Discard?") FALSE ("Discard?") FALSE ("Discard?") FALSE ("Discard?") FALSE ("Discard?") FALSE ("Discard?") w595 w596] -> w528
      event Timeout {
        # "Waits for any of the events to occur"
        n186 = event-data() -> ()  [unwired: 1 in, 1 out]
      }
      event "Top Level folder path": Value Change {
        # "Sends the path specified by the user"
        n187 = event-data() -> ("NewVal"=w539:path)  [unwired: 1 in]
        n188 = To Variant(anything=w539) -> (Variant=w538:variant)
        n189 = Bundle By Name(cluster=T1 {"State"="", "Data"=variant} ("Enqueue Element"), "Data"=w538, "State"="Read Path") -> (w536:T1)
        n190 = Build Array(w536) -> (w535:T1[])
        n191 = call "Queue Driver.vi"("Array of Elements"=w535, "Error In"=w542, "Queue Operation"=Queue_Operation."Enqueue N") -> ("Error Out"=w541:errorcluster)  [unwired: 11 in, 1 out]
      }
      event "Tree": Value Change {
        # "Sends the tags of the selected files and folders"
        n192 = event-data() -> ("NewVal"=w552:string[])  [unwired: 1 in]
        n193 = To Variant(anything=w552) -> (Variant=w547:variant)
        n194 = Bundle By Name(cluster=T1 {"State"="", "Data"=variant} ("Enqueue Element"), "Data"=w547, "State"="Selected Tags") -> (w548:T1)
        n195 = Build Array(w548) -> (w549:T1[])
        n196 = call "Queue Driver.vi"("Array of Elements"=w549, "Error In"=w551, "Queue Operation"=Queue_Operation."Enqueue N") -> ("Error Out"=w550:errorcluster)  [unwired: 11 in, 1 out]
      }
      event "Tree": Mouse Down {
        # "Sends the mouse down co-ordinates"
        n197 = event-data() -> ("Coords"=w563:T6)  [unwired: 1 in]
        n198 = To Variant(anything=w563) -> (Variant=w559:variant)
        n199 = Bundle By Name(cluster=T1 {"State"="", "Data"=variant} ("Enqueue Element"), "Data"=w559, "State"="Trigger Sort") -> (w560:T1)
        n200 = Build Array(w560) -> (w561:T1[])
        n201 = call "Queue Driver.vi"("Array of Elements"=w561, "Error In"=w555, "Queue Operation"=Queue_Operation."Enqueue N") -> ("Error Out"=w554:errorcluster)  [unwired: 11 in, 1 out]
      }
      event "Search Bar": Value Change {
        # "Sends the searched string and performs the expand operation"
        n202 = event-data() -> ("NewVal"=w569:string)  [unwired: 1 in]
        n203 = To Variant(anything=w569) -> (Variant=w574:variant)
        n204 = Bundle By Name(cluster=T1 {"State"="", "Data"=variant} ("Enqueue Element"), "Data"=w574, "State"="Read Search String") -> (w573:T1)
        n205 = Build Array (concatenate)(w573, T1[] [{"State"="Search Results", "Data"=variant}, {"State"="Expand Search", "Data"=variant}] ("appended array")) -> (w572:T1[])
        n206 = call "Queue Driver.vi"("Array of Elements"=w572, "Error In"=w568, "Queue Operation"=Queue_Operation."Enqueue N") -> ("Error Out"=w567:errorcluster)  [unwired: 11 in, 1 out]
      }
      event "Copy": Value Change {
        # "Triggers the copy operation"
        n207 = event-data() -> ()  [unwired: 1 in, 1 out]
        n208 = call "Queue Driver.vi"("Array of Elements"=T1[] [{"State"="Trigger Copy", "Data"=variant}], "Error In"=w576, "Queue Operation"=Queue_Operation."Enqueue N") -> ("Error Out"=w575:errorcluster)  [unwired: 11 in, 1 out]
      }
      event "Expand/Collapse All": Value Change {
        # "Sends the status of the Expand/Collapse boolean"
        n209 = event-data() -> ("NewVal"=w585:bool)  [unwired: 1 in]
        n210 = To Variant(anything=w585) -> (Variant=w588:variant)
        n211 = Bundle By Name(cluster=T1 {"State"="", "Data"=variant} ("Enqueue Element"), "Data"=w588, "State"="Read Expand") -> (w589:T1)
        n212 = Build Array (concatenate)(w589, T1[] [{"State"="Expand or Collapse", "Data"=variant}] ("appended array")) -> (w590:T1[])
        n213 = call "Queue Driver.vi"("Array of Elements"=w590, "Error In"=w584, "Queue Operation"=Queue_Operation."Enqueue N") -> ("Error Out"=w583:errorcluster)  [unwired: 11 in, 1 out]
      }
      event Panel Close? {
        w595 = TRUE ("Discard?")
        # "Triggers the consumer loop to stop and stops the producer"
        n214 = event-data() -> ()  [unwired: 1 in, 1 out]
        n215 = call "Queue Driver.vi"("Array of Elements"=T1[] [{"State"="Exit", "Data"=variant}], "Error In"=w592, "Queue Operation"=Queue_Operation."Enstack N") -> ("Error Out"=w591:errorcluster)  [unwired: 11 in, 1 out]
        n216 = event-data("Discard?"=w595) -> ()  [unwired: 1 in, 1 out]
      }
      event User Event {
        # "Stops the producer loop"
        n217 = event-data() -> ("Stop"=w596:bool)  [unwired: 1 in]
      }
    }
  }
  n218 = Unregister For Events(event registration refnum=w6, error in=w20) -> (error out=w8:errorcluster)
  n219 = Destroy User Event(user event=w2, error in=w8) -> (error out=w7:errorcluster)
  n220 = Merge Errors(w7, w12) -> (→"Error Out":errorcluster)
